vi "Scripting_FindVisOnDiagram.vi"(0 "ViRef":refnum<vi>, 1 "VIsToSerachFor/ViName":variant[](array[variant]), 5 "error in (no error)":errorcluster) -> (15 "VisFound":refnum<vi>[](array[refnum]), 19 "error out":errorcluster)   [LabVIEW 2014]
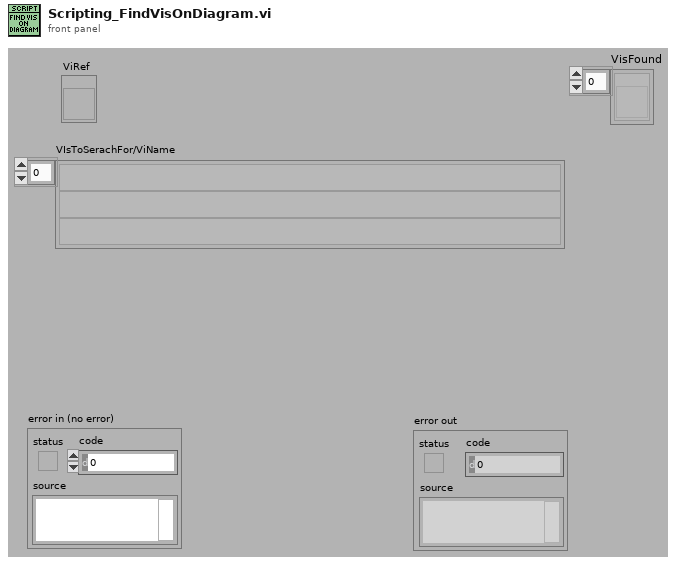
[diagram p1: front panel]
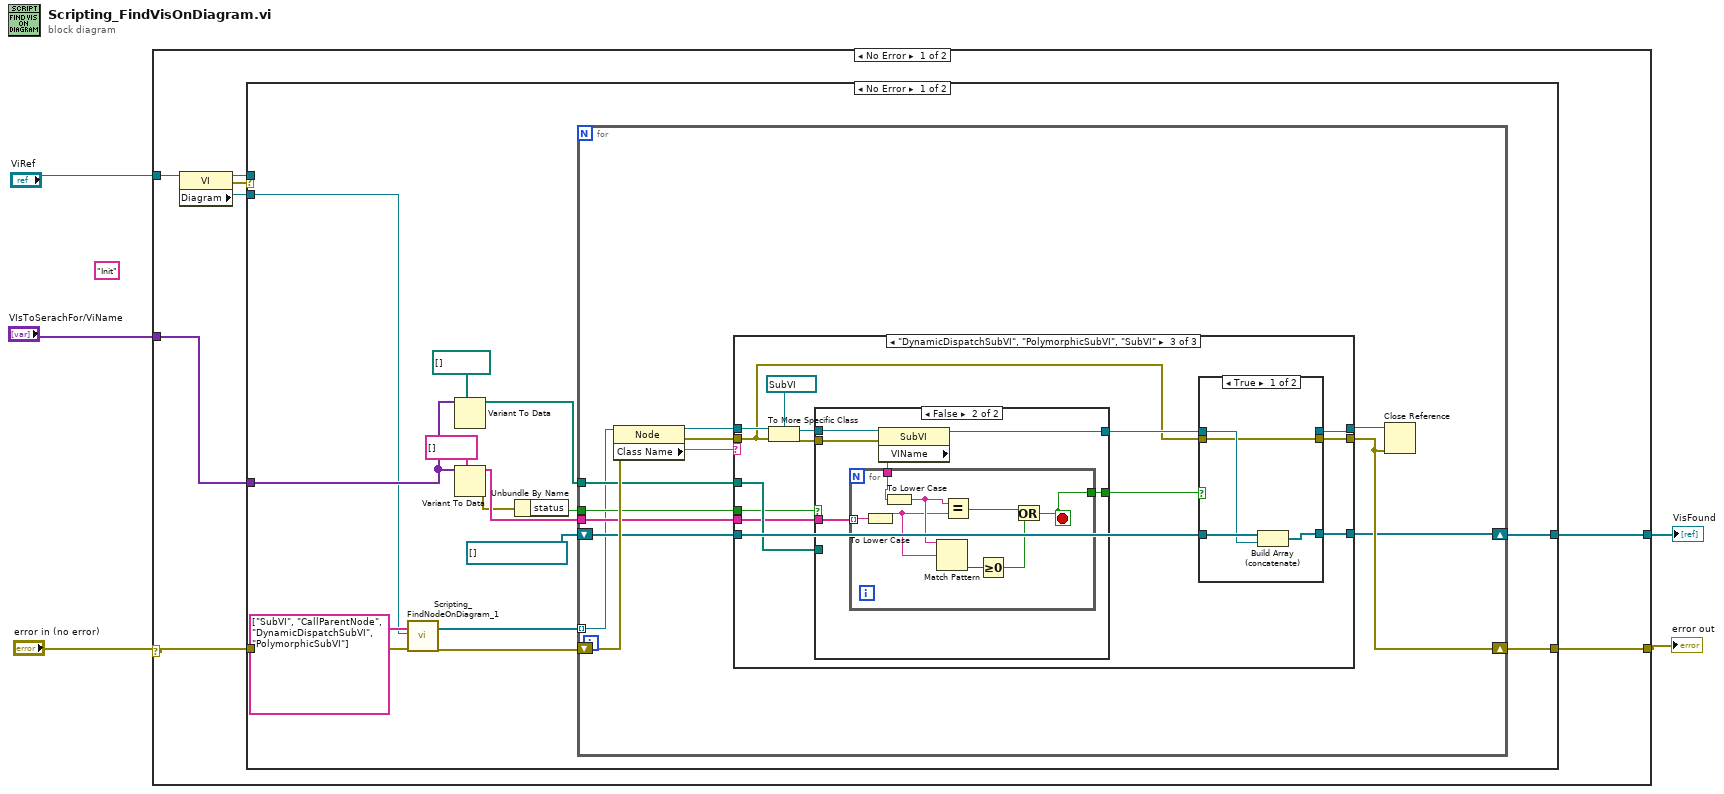
[diagram p0: block diagram]
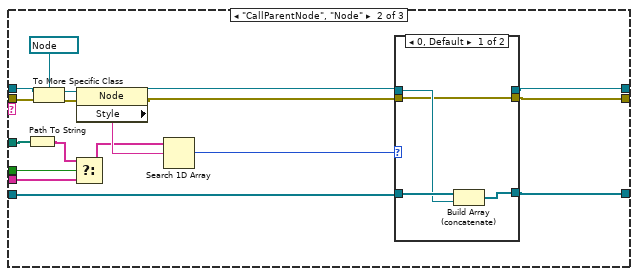
[diagram p3: hidden frame]
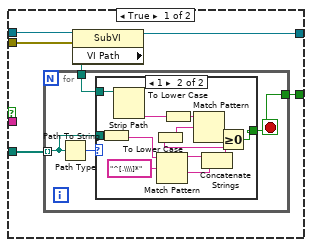
[diagram p5: hidden frame]
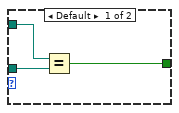
[diagram p6: hidden frame]
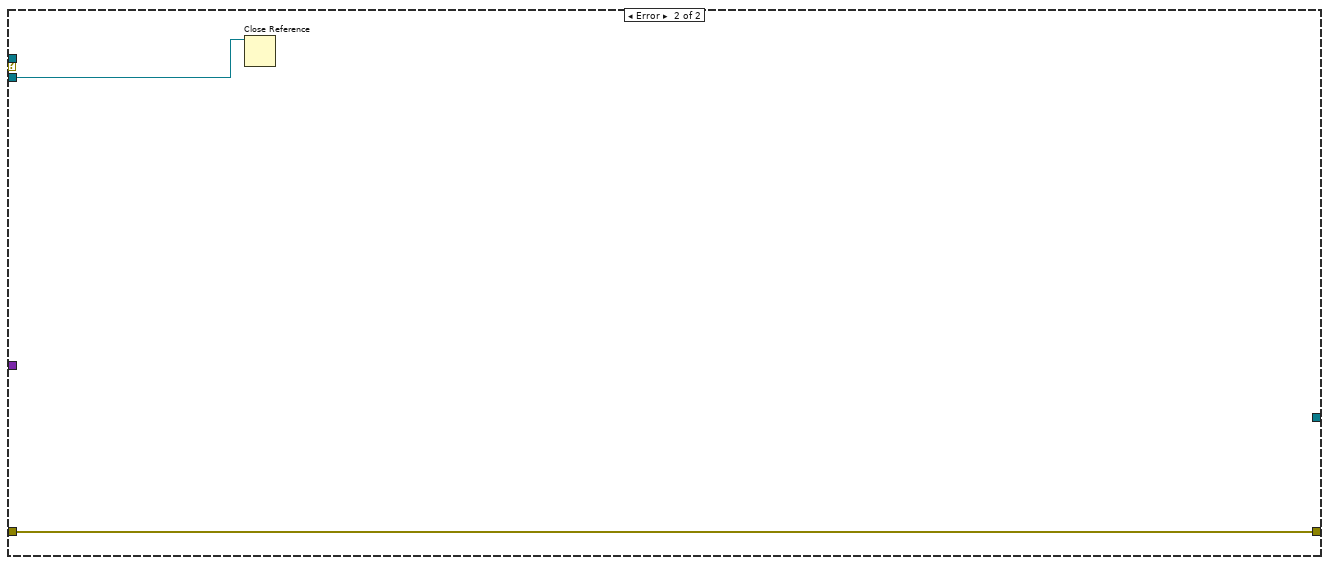
[diagram p8: hidden frame]
diagram:
  (unwired) "Init"
  n1 = case shown="No Error" "error in (no error)" {
    selector: "error in (no error)" -> [w8 w131]
    tunnel: [w13 w131] -> w5
    tunnel: "VIsToSerachFor/ViName" -> [w12 _]
    tunnel: "ViRef" -> [w11 _]
    tunnel: [w7 _] -> w1
    frame No Error {
      n2 = property class="VI"(reference=w11) -> (reference out=w6:refnum<vi>, error out=w9:errorcluster, "Diagram"=w10:refnum<vi>)  [unwired: 1 in]
      n3 = case shown="No Error" w9 {
        tunnel: w10 -> [w15 w129]
        tunnel: [w28 w130] -> w13
        tunnel: w8 -> [w18 w130]
        tunnel: w12 -> [w24 _]
        tunnel: [w26 _] -> w7
        tunnel: w6 -> [_ _]
        frame No Error {
          n4 = call <resource>:"Scripting_FindNodeOnDiagram_1.vi"("NodeTypesToSearchFor"=string[] ["SubVI", "CallParentNode", "DynamicDispatchSubVI", "PolymorphicSubVI"], "Diagram(Ignored If Not Wired)"=w15, "error in (no error)"=w18) -> ("Nodes"=w14:refnum<vi>[], "error out"=w17:errorcluster)  [unwired: 15 in]
          n5 = Variant To Data(type=path[] [] ("VIsToSerachFor/ViName"), Variant=w24) -> (data=w22:path[])  [unwired: 1 in, 1 out]
          n6 = Variant To Data(type=string[] [] ("VIsToSerachFor/ViName"), Variant=w24) -> (data=w21:string[], error out=w20:errorcluster)  [unwired: 1 in]
          n7 = Unbundle By Name(w20) -> ("status"=w19:bool)
          n8 = for {
            shift-right: [w34] -> w28
            shift-left: w17 -> [w36]
            tunnel: w22 -> [w35]
            shift-right: [w32] -> w26
            shift-left: refnum<vi>[] [] -> [w33]
            tunnel: w21 -> [w30]
            tunnel: w19 -> [w31]
            tunnel: w14 -> [w29] mode=indexing
            n9 = property class="Node"(reference=w29, error in=w36) -> (reference out=w39:refnum<vi>, error out=w40:errorcluster, "Class Name"=w38:string)
            n10 = case shown="\"DynamicDispatchSubVI\", \"PolymorphicSubVI\", \"SubVI\"" w38 {
              tunnel: w40 -> [w43 w58 w72]
              tunnel: w39 -> [w42 w59 w82]
              tunnel: [w43 w51 w81] -> w34
              tunnel: [w42 w50 w80] -> w37
              tunnel: w35 -> [_ w57 w73]
              tunnel: w33 -> [w41 w55 w75]
              tunnel: [w41 w52 w74] -> w32
              tunnel: w31 -> [_ w47 w71]
              tunnel: w30 -> [_ w46 w70]
              frame Default {
              }
              frame "CallParentNode", "Node" {
                n11 = Path To String(path=w57) -> (string=w45:string[])
                n12 = To More Specific Class(target class=refnum<vi> refnum ("WhileLoop"), reference=w59, error in=w58) -> (specific class reference=w48:refnum<vi>, error out=w60:errorcluster)
                n13 = Select(t=w45, s=w47, f=w46) -> (s? t:f=w44:string[])
                n14 = property class="Node"(reference=w48, error in=w60) -> (reference out=w53:refnum<vi>, error out=w54:errorcluster, "Style"=w56:string)
                n15 = Search 1D Array(1D array=w44, element=w56) -> (index of element=w49:i32)  [unwired: 1 in]
                n16 = case shown="0, Default" w49 {
                  tunnel: w54 -> [w62 w67]
                  tunnel: w53 -> [w63 w68]
                  tunnel: [_ w68] -> w50
                  tunnel: [w62 w67] -> w51
                  tunnel: w55 -> [w65 w66]
                  tunnel: [w64 w66] -> w52
                  frame 0, Default {
                    n17 = Build Array (concatenate)(w65, w63) -> (w64:refnum<vi>[])
                  }
                  frame -1 {
                  }
                }
              }
              frame "DynamicDispatchSubVI", "PolymorphicSubVI", "SubVI" {
                n18 = To More Specific Class(target class=refnum<vi> refnum ("WhileLoop"), reference=w82, error in=w72) -> (specific class reference=w78:refnum<vi>, error out=w77:errorcluster)
                n19 = case shown="False" w71 {
                  tunnel: w78 -> [w88 w113]
                  tunnel: w77 -> [w87 w112]
                  tunnel: [w86 w111] -> w76
                  tunnel: w73 -> [w85 _]
                  tunnel: [w83 w109] -> w69
                  tunnel: w70 -> [_ w108]
                  frame True {
                    n20 = property class="SubVI"(reference=w88, error in=w87) -> (reference out=w86:refnum<vi>, "VI Path"=w84:path)  [unwired: 1 out]
                    n21 = for {
                      tunnel: w85 -> [w91] mode=indexing
                      tunnel: w84 -> [w90]
                      tunnel: [w89] -> w83
                      stop <- w89 stop-if-true
                      n22 = Path Type(1:w91) -> (0:w92:i16)
                      n23 = case shown="1" w92 {
                        tunnel: w91 -> [w95 w107]
                        tunnel: w90 -> [w94 w106]
                        tunnel: [w93 w103] -> w89
                        frame Default {
                          n24 = Equal?(x=w94, y=w95) -> (x = y?=w93:bool)
                        }
                        frame 1 {
                          n25 = Path To String(path=w107) -> (string=w97:string)
                          n26 = Strip Path(path=w106) -> (name=w105:string)  [unwired: 1 out]
                          n27 = Match Pattern(string=w97, regular expression="^[.\\\\]*") -> (before substring=w99:string, after substring=w98:string)  [unwired: 1 in, 2 out]
                          n28 = To Lower Case(string=w105) -> (all lower case string=w102:string)
                          n29 = Concatenate Strings(w99, w98) -> (w96:string)
                          n30 = To Lower Case(string=w96) -> (all lower case string=w101:string)
                          n31 = Match Pattern(string=w102, regular expression=w101) -> (offset past match=w104:i32)  [unwired: 1 in, 3 out]
                          n32 = Greater Or Equal To 0?(x=w104) -> (x >= 0?=w103:bool)
                        }
                      }
                    }
                  }
                  frame False {
                    n33 = property class="SubVI"(reference=w113, error in=w112) -> (reference out=w111:refnum<vi>, "VIName"=w110:string)  [unwired: 1 out]
                    n34 = for {
                      tunnel: w110 -> [w121]
                      tunnel: [w114] -> w109
                      tunnel: w108 -> [w120] mode=indexing
                      stop <- w114 stop-if-true
                      n35 = To Lower Case(string=w120) -> (all lower case string=w117:string)
                      n36 = To Lower Case(string=w121) -> (all lower case string=w118:string)
                      n37 = Match Pattern(string=w118, regular expression=w117) -> (offset past match=w116:i32)  [unwired: 1 in, 3 out]
                      n38 = Equal?(x=w118, y=w117) -> (x = y?=w119:bool)
                      n39 = Greater Or Equal To 0?(x=w116) -> (x >= 0?=w115:bool)
                      n40 = Or(x=w119, y=w115) -> (x .or. y?=w114:bool)
                    }
                  }
                }
                n41 = case shown="True" w69 {
                  tunnel: w72 -> [w122 w127]
                  tunnel: w76 -> [w123 w128]
                  tunnel: [_ w128] -> w80
                  tunnel: [w122 w127] -> w81
                  tunnel: w75 -> [w125 w126]
                  tunnel: [w124 w126] -> w74
                  frame True {
                    n42 = Build Array (concatenate)(w125, w123) -> (w124:refnum<vi>[])
                  }
                  frame False {
                  }
                }
              }
            }
            n43 = Close Reference(reference=w37, error in (no error)=w34) -> ()  [unwired: 1 out]
          }
        }
        frame Error {
          n44 = Close Reference(reference=w129) -> ()  [unwired: 1 in, 1 out]
        }
      }
    }
    frame Error {
    }
  }
  "error out" <- w5
  "VisFound" <- w1
